vi "Write RIO FPGA.vi"(8 "error in":errorcluster, 10 "RIO FPGA":string, 11 "PL_Target Configuration in":refnum<class "PL_Target Configuration.lvclass">) -> (0 "error out":errorcluster, 3 "PL_Target Configuration out":refnum<class "PL_Target Configuration.lvclass">)   [LabVIEW 2013, in "PL_Target Configuration.lvclass"]
uses:
  PL_Target Configuration.lvclass
  PL_Target Configuration.lvclass/PL_Target Configuration.ctl
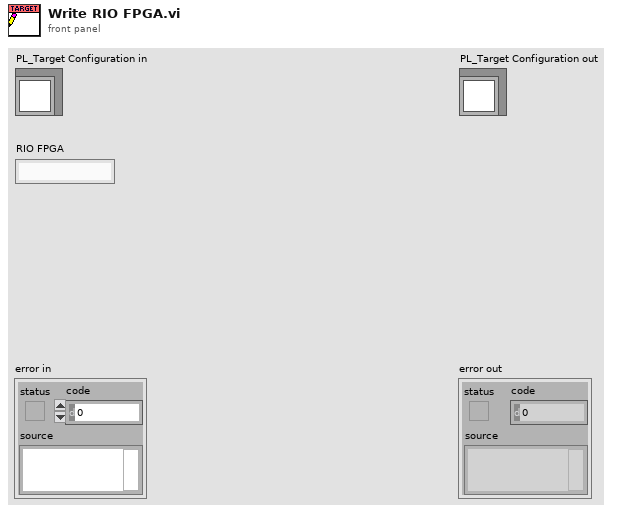
[diagram p1: front panel]
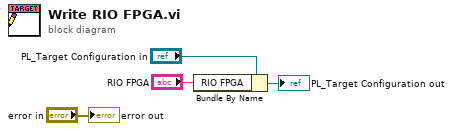
[diagram p0: block diagram]
diagram:
  n1 = Bundle By Name(cluster="PL_Target Configuration in", "RIO FPGA"="RIO FPGA") -> (→"PL_Target Configuration out":refnum<class "PL_Target Configuration.lvclass">)
  "error out" <- "error in"
